vi "Configure Digital Gen Arbitrary Waveform.vi"(0 "VISA resource name":refnum<visa-resource-name>, 1 "Output Rate (10 %)":dbl=10.0, 2 "Column Select (0)":i32, 5 "Channel (0: chA)":i32(ring) items=["chA", "chB"], 7 "Amplitude (0 FFS)":dbl, 9 "Enable Over Sampling (T: Enable)":bool=TRUE, 11 "error in (no error)":errorcluster, 12 "Load File (\"MyFile.arb\")":string="\"MyFile.arb\"", 13 "Enable Waveform (T: Enable)":bool=TRUE) -> (4 "VISA resource name out":refnum<visa-resource-name>, 15 "error out":errorcluster)   [LabVIEW 2014, in "Stanford Research SR1.lvlib"]
doc: "Configures the attributes for the Digital Generator Arbitrary Waveform."
uses:
  Stanford Research SR1.lvlib
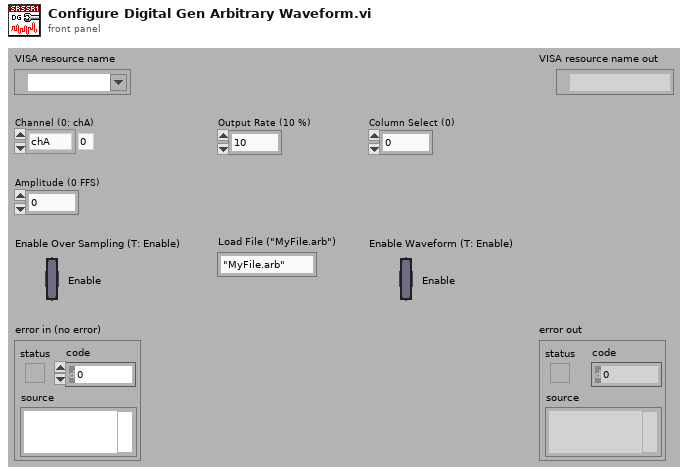
[diagram p1: front panel]
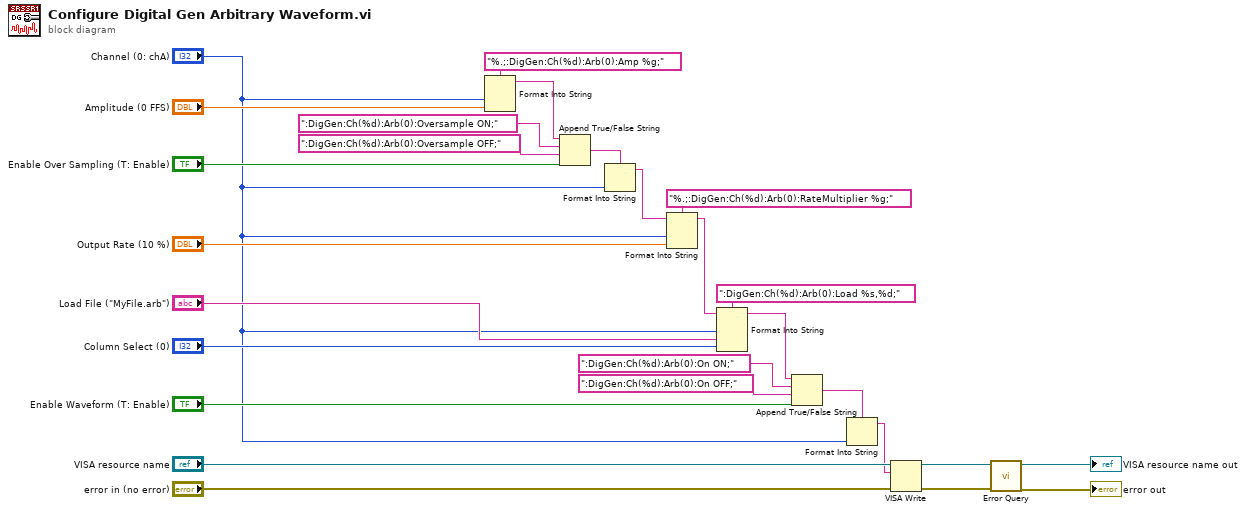
[diagram p0: block diagram]
diagram:
  n1 = Format Into String(format string="%.;:DigGen:Ch(%d):Arb(0):Amp %g;", "Channel (0: chA)", "Amplitude (0 FFS)") -> (resulting string=w26:string)  [unwired: 2 in, 1 out]
  n2 = Append True/False String(1:"Enable Over Sampling (T: Enable)", 2:":DigGen:Ch(%d):Arb(0):Oversample OFF;", 3:":DigGen:Ch(%d):Arb(0):Oversample ON;", 4:w26) -> (0:w3:string)
  n3 = Format Into String(format string=w3, "Channel (0: chA)") -> (resulting string=w2:string)  [unwired: 2 in, 1 out]
  n4 = Format Into String(format string="%.;:DigGen:Ch(%d):Arb(0):RateMultiplier %g;", initial string=w2, "Channel (0: chA)", "Output Rate (10 %)") -> (resulting string=w21:string)  [unwired: 1 in, 1 out]
  n5 = Format Into String(format string=":DigGen:Ch(%d):Arb(0):Load %s,%d;", initial string=w21, "Channel (0: chA)", "Load File (\"MyFile.arb\")", "Column Select (0)") -> (resulting string=w19:string)  [unwired: 1 in, 1 out]
  n6 = Append True/False String(1:"Enable Waveform (T: Enable)", 2:":DigGen:Ch(%d):Arb(0):On OFF;", 3:":DigGen:Ch(%d):Arb(0):On ON;", 4:w19) -> (0:w5:string)
  n7 = Format Into String(format string=w5, "Channel (0: chA)") -> (resulting string=w4:string)  [unwired: 2 in, 1 out]
  n8 = VISA Write(VISA resource name="VISA resource name", write buffer=w4, error in (no error)="error in (no error)") -> (VISA resource name out=w13:refnum<visa-resource-name>, error out=w12:errorcluster)  [unwired: 1 out]
  n9 = call "Error Query.vi"("error in (no error)"=w12, "VISA resource name"=w13) -> ("error out"=→"error out":errorcluster, "VISA resource name out"=→"VISA resource name out":refnum<visa-resource-name>)  [unwired: 6 in, 2 out]
